vi "Clear Sequence Table Results.vi"(8 "error in (no error)":errorcluster, 11 "table reference in":refnum<vi>) -> (0 "error out":errorcluster, 3 "table reference out":refnum<vi>)   [LabVIEW 2019, in "View Reports.lvlib"]
uses:
  View Reports.lvlib
  <vilib>/Utility/miscctls.llb/LVRowAndColumnTypeDef.ctl
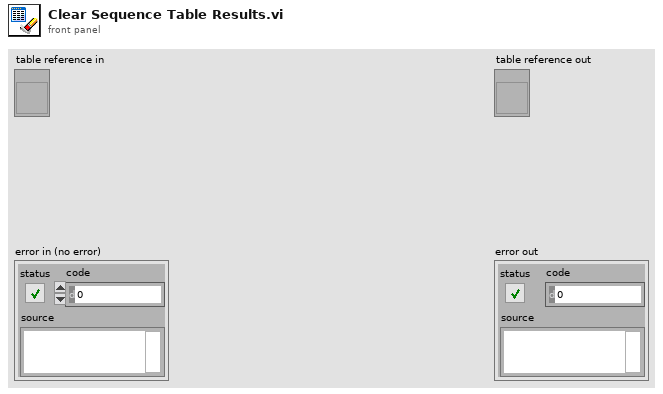
[diagram p1: front panel]
types:
  T1 = typedef "LVRowAndColumnTypeDef.ctl" = cluster{"Row":i32, "Column":i32}
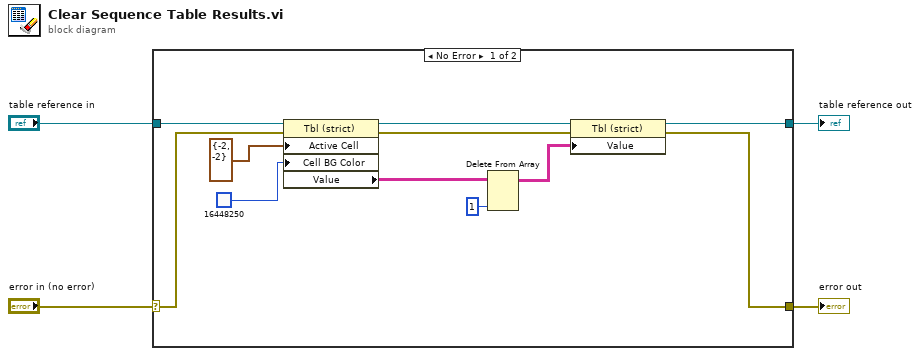
[diagram p0: block diagram]
diagram:
  n1 = case shown="No Error" "error in (no error)" {
    selector: "error in (no error)" -> [w8 w17]
    tunnel: "table reference in" -> [w15 w16]
    tunnel: [w6 w17] -> w2
    tunnel: [w5 w16] -> w1
    frame No Error {
      n2 = property class="Tbl (strict)"(reference=w15, error in=w8, "Active Cell"=T1 {"Row"=-2, "Column"=-2} ("Active Cell:Active Cell"), "Cell BG Color"=u32 16448250) -> (reference out=w12:refnum<vi>, error out=w7:errorcluster, "Value"=w11:string[][])
      n3 = Delete From Array(array=w11, index (col)=1 ("disabled index (col)")) -> (array with subset deleted=w9:string[][])  [unwired: 2 in, 1 out]
      n4 = property class="Tbl (strict)"(reference=w12, error in=w7, "Value"=w9) -> (reference out=w5:refnum<vi>, error out=w6:errorcluster)
    }
    frame Error {
    }
  }
  "error out" <- w2
  "table reference out" <- w1
